vi "delta_wieksza_zero.vi"(10 "delta":dbl, 11 "q":dbl) -> (3 "y0":dbl)   [LabVIEW 2020]
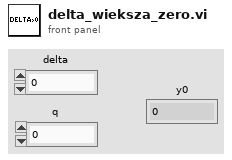
[diagram p1: front panel]
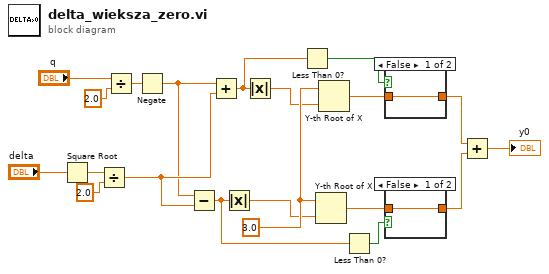
[diagram p0: block diagram]
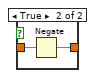
[diagram p2: hidden frame]
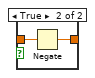
[diagram p3: hidden frame]
diagram:
  w20 = 3.0 ("x")
  n1 = Square Root(x="delta") -> (sqrt(x)=w16:dbl)
  n2 = Divide(x=w16, y=2.0) -> (x/y=w19:dbl)
  n3 = Divide(x="q", y=2.0) -> (x/y=w17:dbl)
  n4 = Negate(x=w17) -> (-x=w18:dbl)
  n5 = Subtract(x=w18, y=w19) -> (x-y=w8:dbl)
  n6 = Add(x=w18, y=w19) -> (x+y=w2:dbl)
  n7 = Absolute Value(x=w8) -> (abs(x)=w10:dbl)
  n8 = Absolute Value(x=w2) -> (abs(x)=w9:dbl)
  n9 = Less Than 0?(x=w2) -> (x < 0?=w1:bool)
  n10 = Y-th Root of X(1:w10, 2:w20) -> (0:w7:dbl)
  n11 = Y-th Root of X(1:w9, 2:w20) -> (0:w4:dbl)
  n12 = Less Than 0?(x=w8) -> (x < 0?=w5:bool)
  n13 = case shown="False" w1 {
    tunnel: w4 -> [w21 w23]
    tunnel: [w21 w22] -> w3
    frame False {
    }
    frame True {
      n14 = Negate(x=w23) -> (-x=w22:dbl)
    }
  }
  n15 = case shown="False" w5 {
    tunnel: w7 -> [w24 w26]
    tunnel: [w24 w25] -> w6
    frame False {
    }
    frame True {
      n16 = Negate(x=w26) -> (-x=w25:dbl)
    }
  }
  n17 = Add(x=w3, y=w6) -> (x+y=→"y0":dbl)
